vi "sin.vi"(8 "error constant":errorcluster, 10 "noise amplitude":dbl, 11 "dx":dbl) -> (0 "error constant 2":errorcluster, 3 "sin x":dbl)   [LabVIEW 2022 SP3]
uses:
  <vilib>/numeric/Random Number (Range) DBL.vi
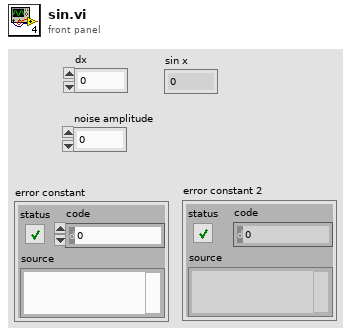
[diagram p1: front panel]
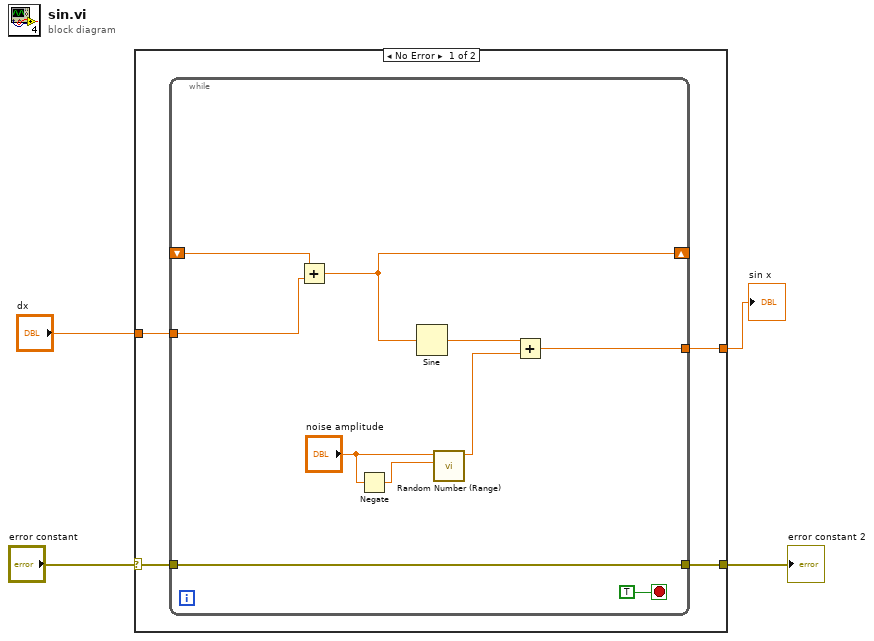
[diagram p0: block diagram]
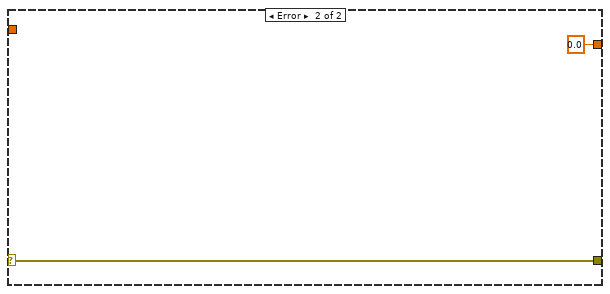
[diagram p2: hidden frame]
diagram:
  n1 = case shown="No Error" "error constant" {
    selector: "error constant" -> [w7 w20]
    tunnel: "dx" -> [w8 _]
    tunnel: [w6 w20] -> w2
    tunnel: [w5 0.0] -> w1
    frame No Error {
      n2 = while {
        shift-right: [w14] -> _
        shift-left: _ -> [w17]
        tunnel: w8 -> [w16]
        tunnel: [w15] -> w6
        tunnel: w7 -> [w15]
        tunnel: [w12] -> w5
        stop <- TRUE stop-if-true
        n3 = Add(x=w17, y=w16) -> (x+y=w14:dbl)
        n4 = Negate(x="noise amplitude") -> (-x=w9:dbl)
        n5 = Sine(x=w14) -> (sin(x)=w13:dbl)
        n6 = call-poly <vilib>:"Random Number (Range).vi"("lower bound (0)"=w9, "upper bound (100)"="noise amplitude") -> ("number"=w11:dbl)  [unwired: 9 in]
        n7 = Add(x=w13, y=w11) -> (x+y=w12:dbl)
      }
    }
    frame Error {
    }
  }
  "error constant 2" <- w2
  "sin x" <- w1
